vi "TLB Native Dynamic Events ver 0.06b.vi"() -> ()   [LabVIEW 2018]
uses:
  Labview Training Phase 2/Enum Controls/States for Action Engine.ctl
  Type def/TLB event states.ctl
  Type def/TLB MHL States.ctl
  <vilib>/Studica/Studica Toolkit/Background/I2C Channel.ctl
  <vilib>/Studica/Studica Toolkit/NavX/NavX.lvlib
  <vilib>/myRIO/Common/Instrument Driver Framework/myRIO v1.0/AI/typedefs/AI Channels Enum.ctl
  <vilib>/myRIO/Common/Instrument Driver Framework/myRIO v1.0/AI/typedefs/AI Channels List.ctl
  Type def/Type def.ctl
  Type def/Motor Control Cluster.ctl
  <vilib>/Studica/Studica Blackhawk/Blackhawk.lvlib
  <vilib>/vision/driver/NI_Vision_Acquisition_Software.lvlib
  <vilib>/userdefined/High Color/IMAQdx.ctl
  <vilib>/vision/driver/IMAQdx.llb/IMAQdx Buffer Number Mode.ctl
  <vilib>/vision/driver/IMAQdx.llb/IMAQdx Acquisition Mode.ctl
  Underlying VI's/Webcam FGV Low level ver/State control.ctl
  <vilib>/Studica/Studica Toolkit/Background/Mxp Selection.ctl
  <vilib>/ptbypt/NI_PtbyPt.lvlib
panel:
  out "Speed and distance cluster":T1
  out "error out":errorcluster
  out "Blackhawk loop":i32
  out "NavX Loop":i32
  out "Sensor Loop":i32
  out "User event loop":i32
  out "Event handling loop":i32
  out "Main Loop":i32
  out "Status loop":i32
  out "L/R average":fxp<+,64,64>
  out "Right Ultrasonic":fxp<+,64,16>
  out "Left Ultrasonic":fxp<+,64,16>
  out "Object detection count":T2
  out "Camera error":errorcluster
  out "Right IR Sensor":dbl
  out "Left IR Sensor":dbl
  in  "Servo Angle":u8(slide) scale=0.0..180.0
  in  "On/Off":bool
  out "Blackhawk error":errorcluster
  out "Value Read":bool
  out "Image Out":T3(plugin-control)
  out "element":T4
  out "Action Queue Items":i32
  out "State Logic Queue Items":i32
  out "Action Queues items":string[](array[string])=["Hardware reset", "Software reset", ""]
  out "State logic":T5=enum."Task 2"
  out "Action State":string
  in  "Tasks Selector":string(combo)="Default"
  out "Yaw":dbl
  out "NavX Info Out":T7
  out "LinearAcceleration":T8
  out "Displacement":T9
  out "YRPHfH":T10
  out "Object detected":bool
  in  "NavX Zero Yaw":bool
  in  "Return to IDLE":bool
  in  "Stop Queue":bool
  in  "Start Task":bool
  # "Camera Status Loop"
  # "TLB FRAMEWORK STATUS"
  # "Test Programme written by Calvin Loke    Dated: 28 Aug 2019\nTest Programme revised by Dr Alex See   Dated 30 Aug 2019\n\nProgramme version:   TLB Native Dynamic Events ver 0.04b.vi"
  # "Sequence of Actions"
  # "Continuous (Repeated)"
  # "Motor Control Loop"
  # "Sensor data"
  # "Blackhawk status"
  # "System Health Status Update"
  # "NAVX Control Loop"
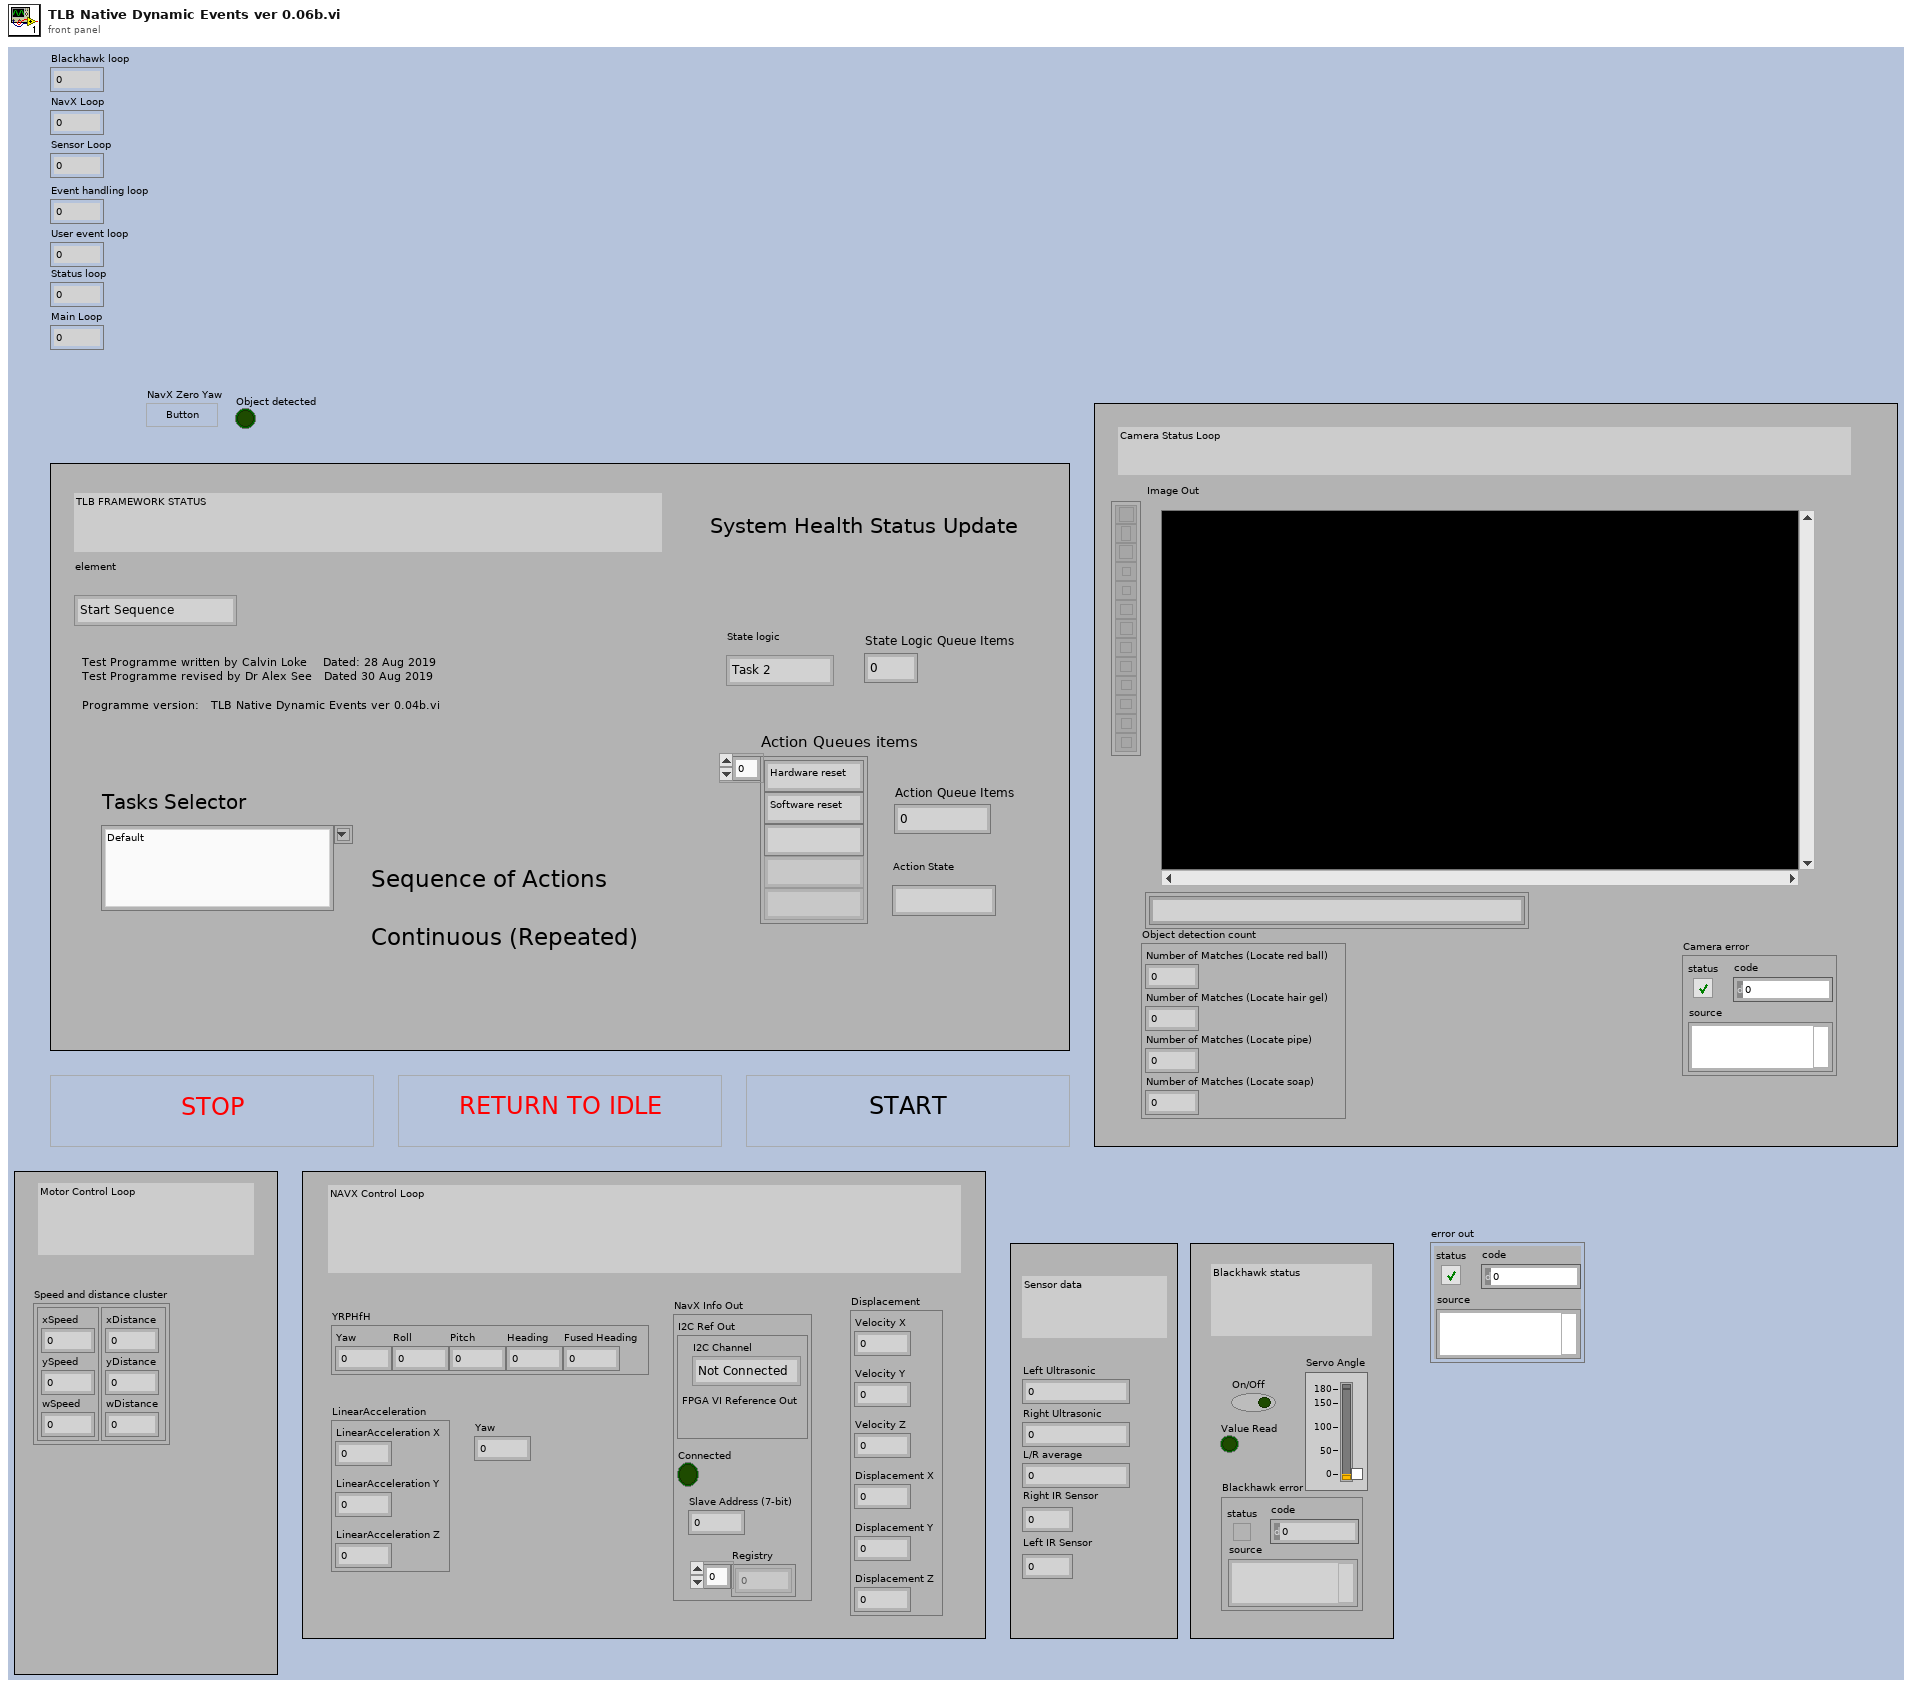
[diagram p1: front panel]
types:
  T1 = cluster{cluster{"xSpeed":dbl, "ySpeed":dbl, "wSpeed":dbl}, cluster{"xDistance":dbl, "yDistance":dbl, "wDistance":dbl}}
  T2 = cluster{"Number of Matches (Locate red ball)":i32, "Number of Matches (Locate hair gel)":i32, "Number of Matches (Locate pipe)":i32, "Number of Matches (Locate soap)":i32}
  T3 = typedef "IMAQ Image.ctl" = refnum<image>
  T4 = typedef "TLB event states.ctl" = enum16{"Start Sequence", "Exit", "Start Task 1", "Start Task 2", "Start Task 3", "Start Task 4", "Camera vision", "Wall follow mode", "Idle", "Start Drive Straight"}
  T5 = typedef "TLB MHL States.ctl" = enum16{"None", "Startup", "Idle", "Processing", "Shutdown", "Reset", "Task 1", "Task 2", "Task 3", "Task 4", "Task 4a", "Task 4b", "Task 4c", "Task 4d", "Task 4e", "Task 4f", "Task 4g", "Task 4h", "Acquire image", "Wall follow mode", "Autodrive", "Autodrive a"}
  T6 = typedef "I2C Channel.ctl" = enum16{"Not Connected", "A", "B"}
  T7 = cluster{"I2C Ref Out":cluster{"I2C Channel":T6, "FPGA VI Reference Out":refnum<k20>}, "Connected":bool, "Slave Address (7-bit)":u8, "Registry":u8[]}
  T8 = cluster{"LinearAcceleration X":dbl, "LinearAcceleration Y":dbl, "LinearAcceleration Z":dbl}
  T9 = cluster{"Velocity X":dbl, "Velocity Y":dbl, "Velocity Z":dbl, "Displacement X":dbl, "Displacement Y":dbl, "Displacement Z":dbl}
  T10 = cluster{"Yaw":dbl, "Roll":dbl, "Pitch":dbl, "Heading":dbl, "Fused Heading":dbl}
  T11 = typedef "States for Action Engine.ctl" = enum16{"Initialize", "Write", "Read"}
  T12 = typedef "Motor Control Cluster.ctl" = cluster{"Vx":dbl, "Vy":dbl, "Vw":dbl}
  T13 = typedef "Type def.ctl" = cluster{"Front Ultrasonic Obstruct":bool, "Left Ultrasonic Obstruct":bool, "Right Ultrasonic Obstruct ":bool}
  T14 = typedef "NI_Vision_Acquisition_Software.lvlib/IMAQdx Acquisition Mode.ctl" = enum32{"One Shot", "Continuous"}
  T15 = typedef "IMAQdx.ctl" = refnum<k21>
  T16 = typedef "NI_Vision_Acquisition_Software.lvlib/IMAQdx Buffer Number Mode.ctl" = enum32{"Next", "Last", "Buffer Number", "Every", "Last New"}
  T17 = typedef "Mxp Selection.ctl" = enum16{"MXP A", "MXP B"}
  T18 = cluster{"xTargetSpeed":dbl, "yTargetSpeed":dbl, "wTargetSpeed":dbl}
  T19 = typedef "State control.ctl" = enum16{"Initialise", "Start camera", "Continuous Acquisition ", "Stop camera", "Dispose all"}
  T20 = cluster{"xDistance":dbl, "yDistance":dbl, "wDistance":dbl}
  T21 = typedef "AI Channels List.ctl" = T22[]
  T22 = typedef "AI Channels Enum.ctl" = enum16{"Not Connected", "AudioIn/Left", "AudioIn/Right", "C/AI0", "C/AI1", "A/AI0", "A/AI1", "A/AI2", "A/AI3", "A/AI4", "A/AI5", "A/AI6", "A/AI7", "B/AI0", "B/AI1", "B/AI2", "B/AI3", "B/AI4", "B/AI5", "B/AI6", "B/AI7", "AI/AI0", "AI/AI1", "AI/AI2", "AI/AI3", "A/AI0 (DIFF)", "A/AI1 (DIFF)", "A/AI2 (DIFF)", "A/AI3 (DIFF)", "B/AI0 (DIFF)", "B/AI1 (DIFF)", "B/AI2 (DIFF)", "B/AI3 (DIFF)"}
  T23 = cluster{"I2C Channel":T6, "FPGA VI Reference Out":refnum<k20>}
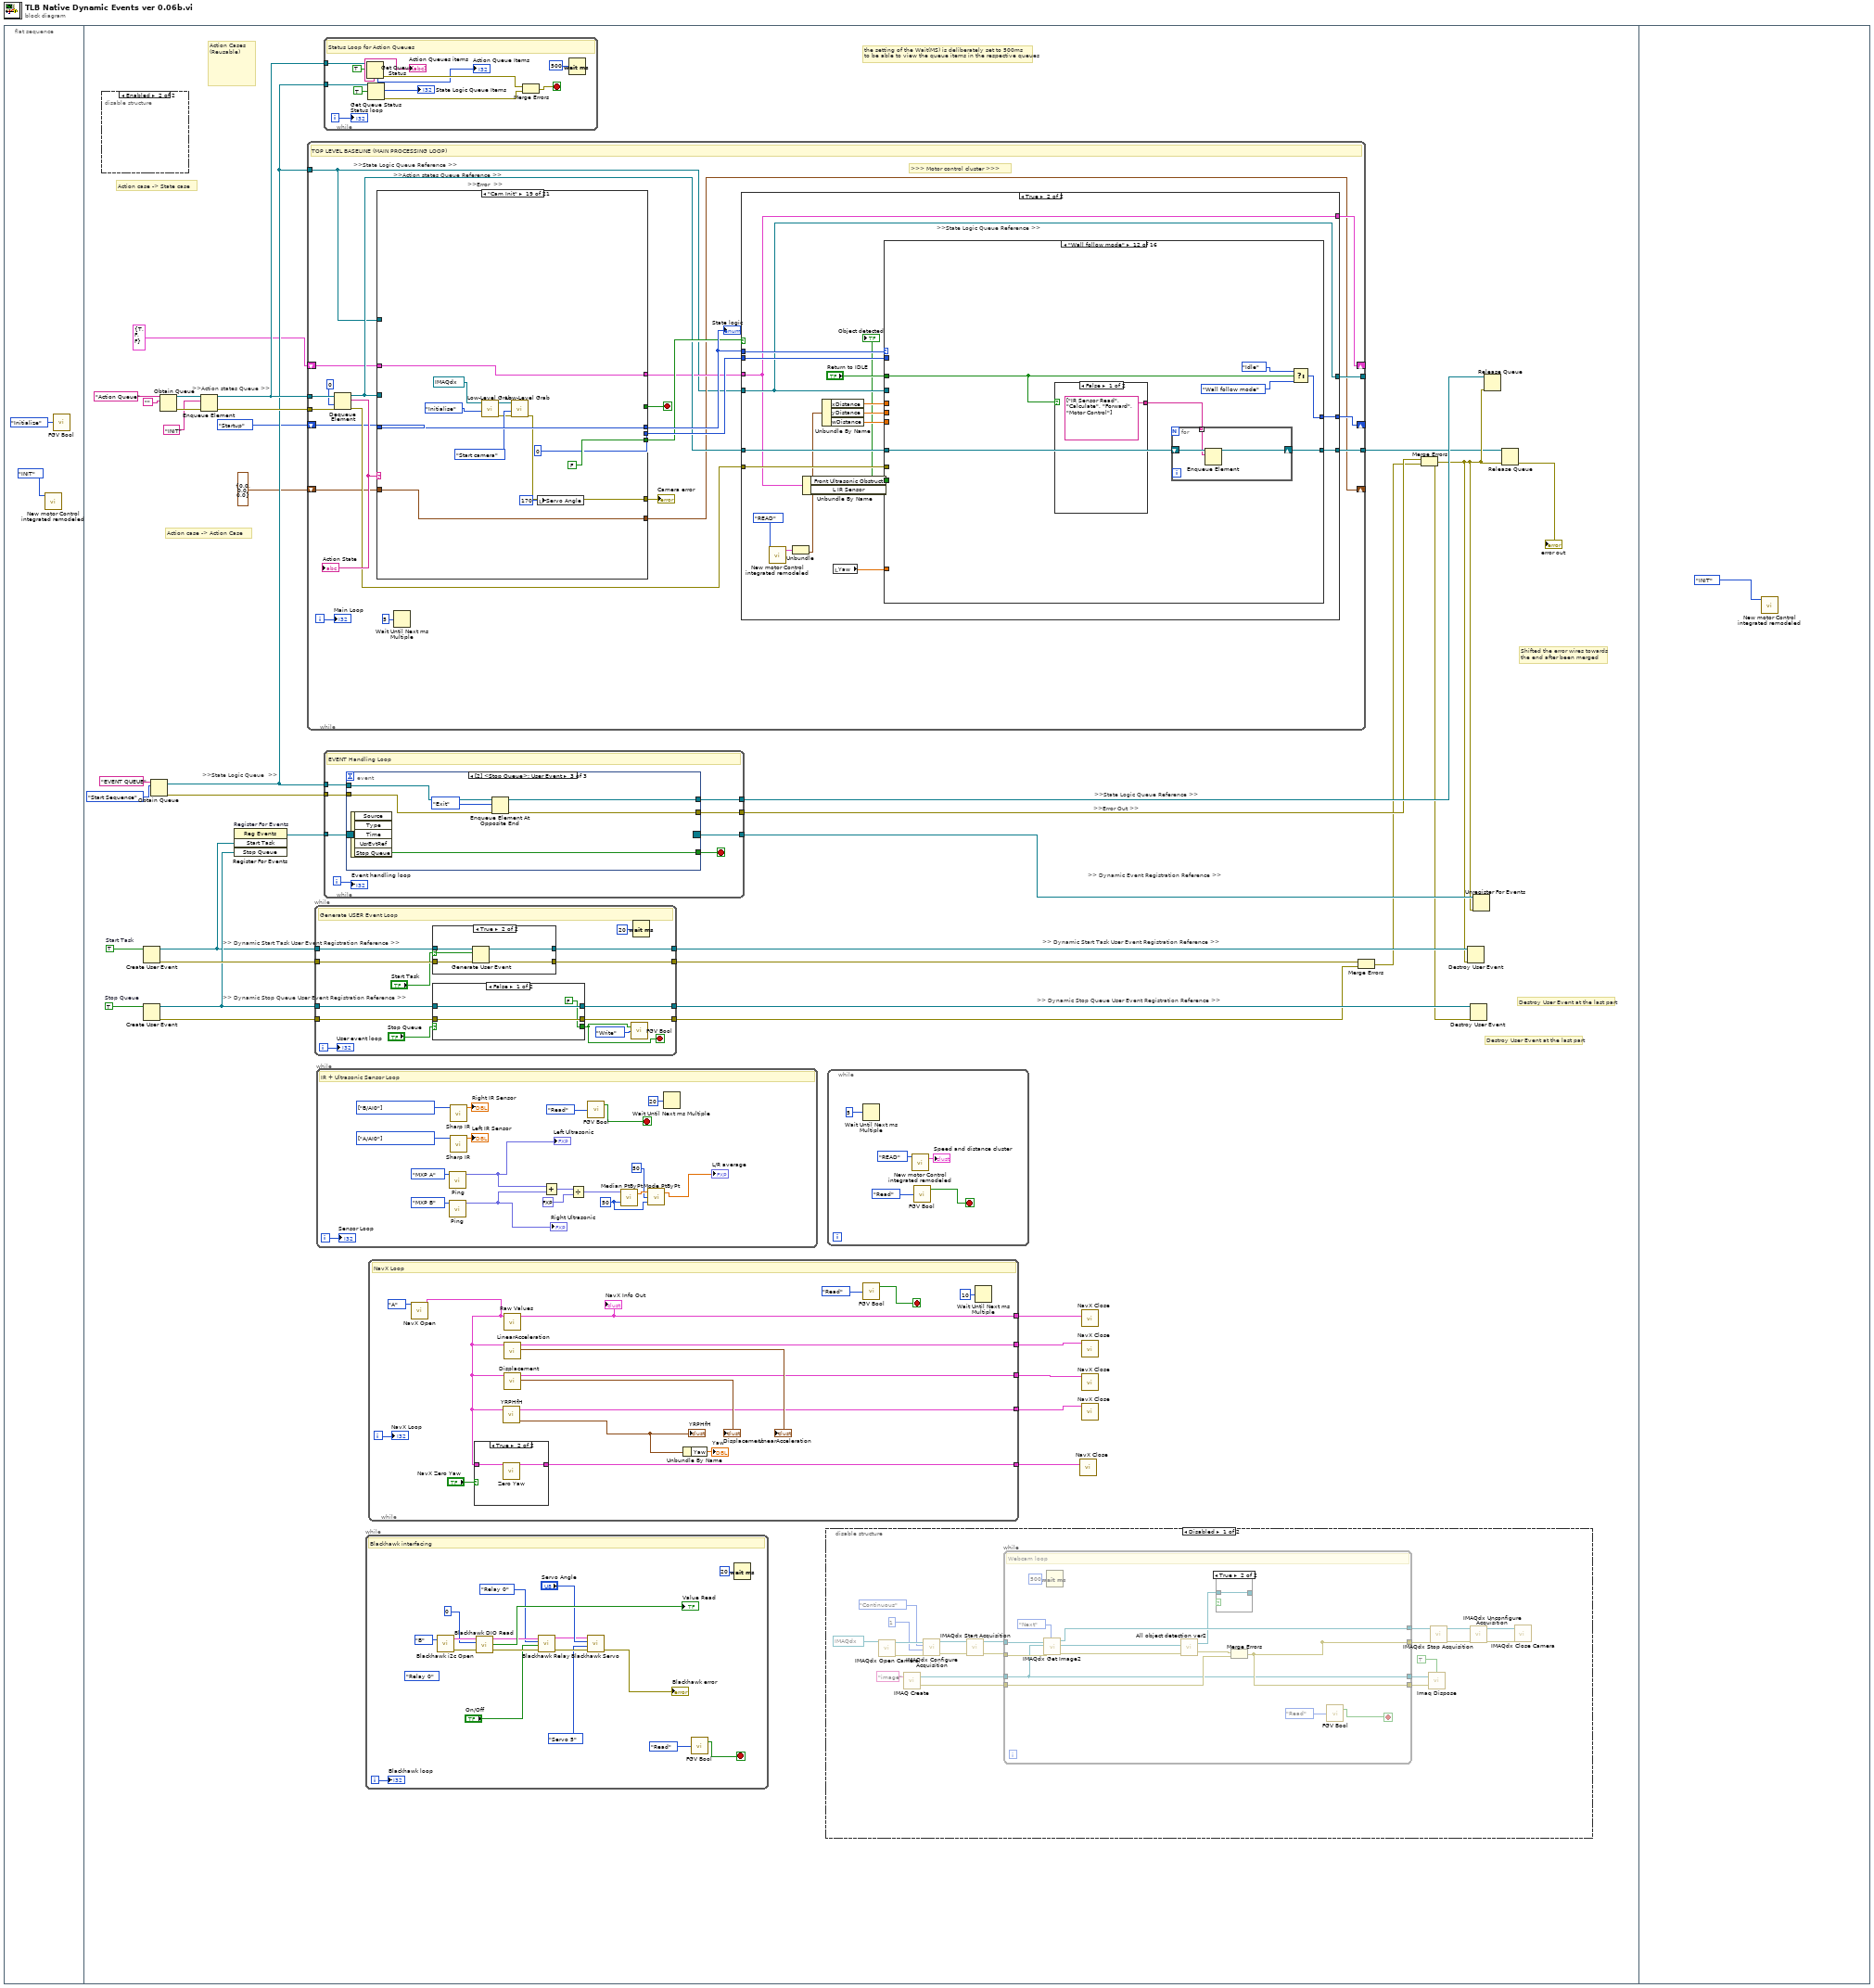
[diagram p0: block diagram]
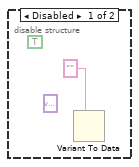
[diagram p5: hidden frame]
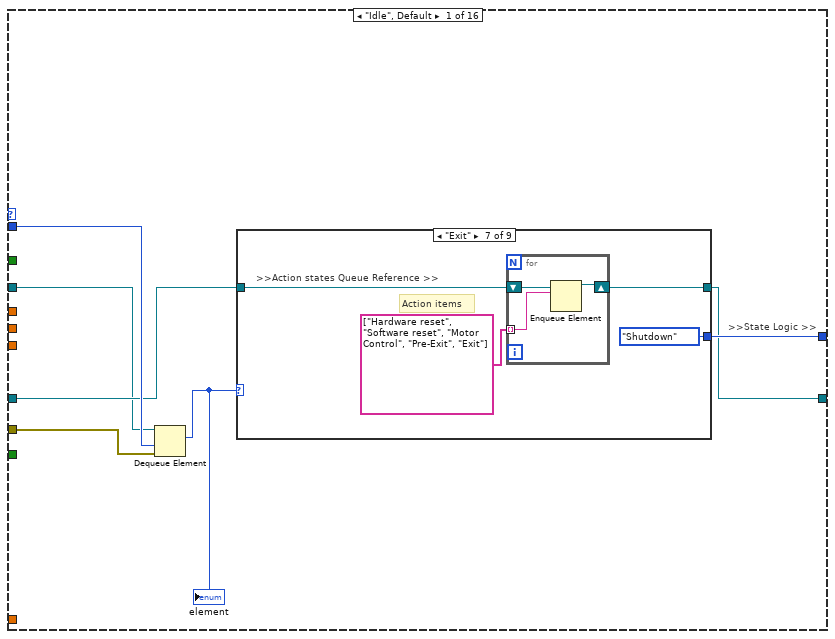
[diagram p7: hidden frame]
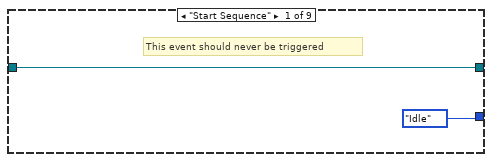
[diagram p8: hidden frame]
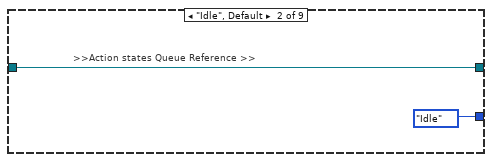
[diagram p9: hidden frame]
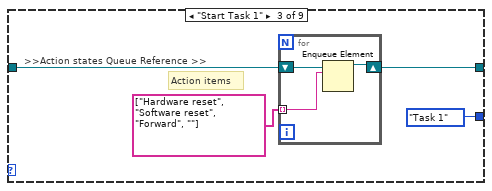
[diagram p10: hidden frame]
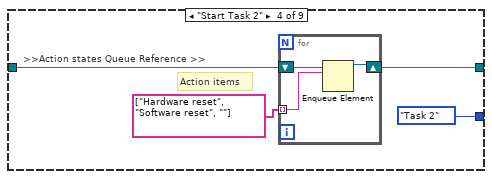
[diagram p11: hidden frame]
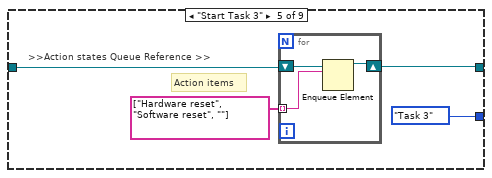
[diagram p12: hidden frame]
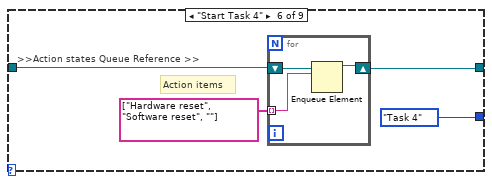
[diagram p13: hidden frame]
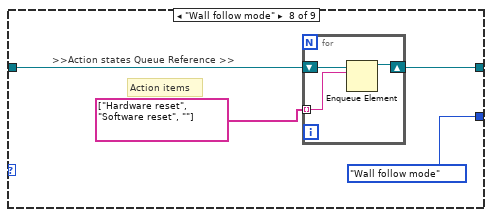
[diagram p14: hidden frame]
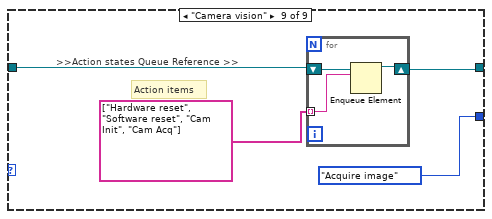
[diagram p15: hidden frame]
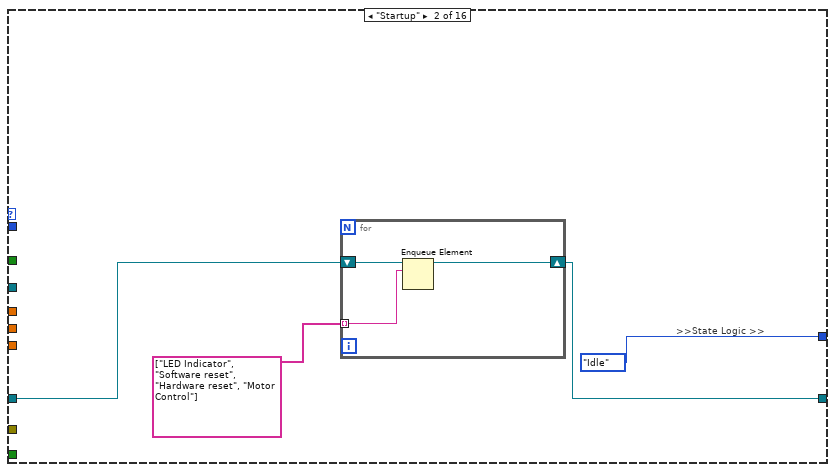
[diagram p16: hidden frame]
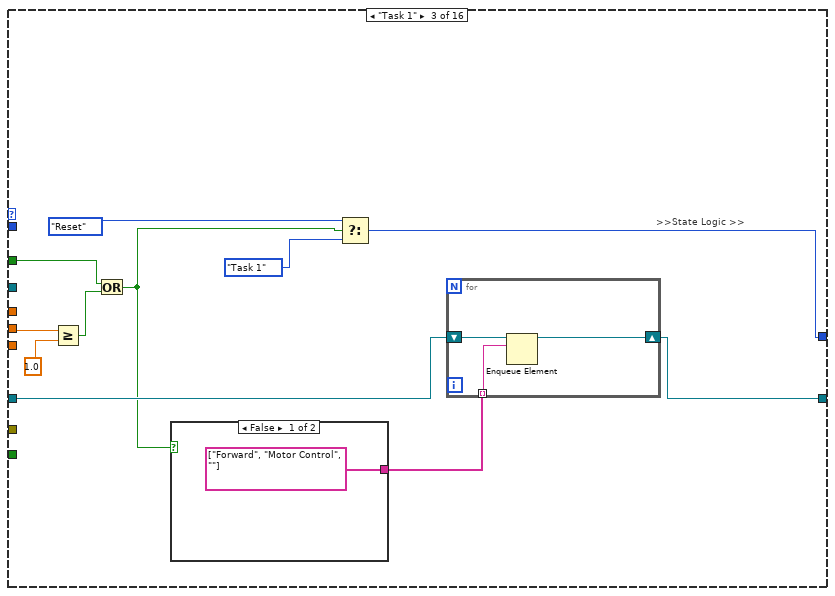
[diagram p17: hidden frame]
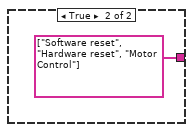
[diagram p18: hidden frame]
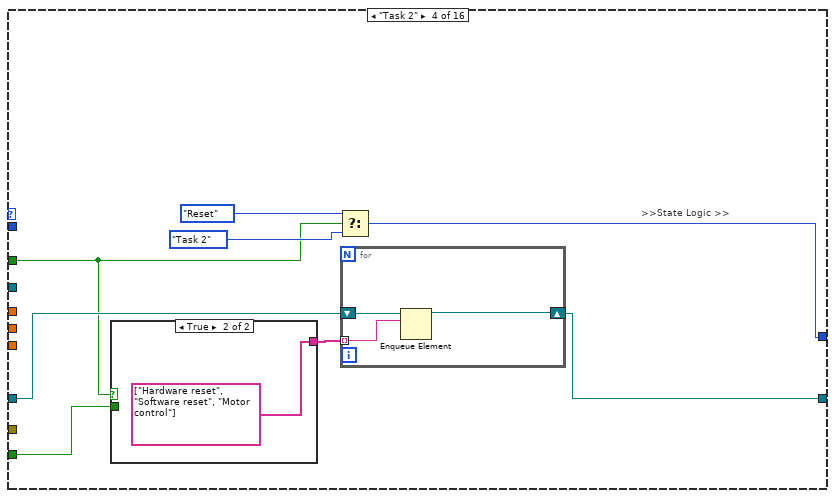
[diagram p19: hidden frame]
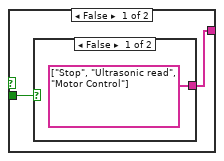
[diagram p20: hidden frame]
diagram:
  n1 = flat-sequence {
    frame #0 {
      n2 = call "New motor Control integrated remodeled.vi"("States"=enum16{"RESET ENCODER", "WRITE", "READ", "INIT"}."INIT") -> ()  [unwired: 4 in, 2 out]
      n3 = call "FGV Bool.vi"("Init/Read/Write State"=States_for_Action_Engine."Initialize") -> ()  [unwired: 2 in, 2 out]
    }
    frame #1 {
      w38 = TRUE  # Stop Queue
      w37 = TRUE  # Start Task
      # "Action case -> Action Case"
      # "Action case -> State case"
      # "the setting of the Wait(MS) is deliberately set to 500ms\nto be able to view the queue items in the respective queues"
      # "Action Cases\n(Reusable)"
      # ">>Error Out >>"
      # ">> Dynamic Stop Queue User Event Registration Reference >>"
      # ">> Dynamic Start Task User Event Registration Reference >>"
      # ">> Dynamic Stop Queue User Event Registration Reference >>"
      # ">> Dynamic Start Task User Event Registration Reference >>"
      # ">> Dynamic Event Registration Reference >>"
      # ">>Action states Queue >>"
      # ">>State Logic Queue  >>"
      # ">>State Logic Queue Reference >>"
      # "Destroy User Event at the last part"
      # "Destroy User Event at the last part"
      # "Shifted the error wires towards\nthe end after been merged"
      n4 = disable-structure shown="Enabled" {
        frame Disabled {
          (unwired) variant
          (unwired) TRUE
          n5 = Variant To Data(type="") -> ()  [unwired: 2 in, 2 out]
        }
        frame Enabled {
        }
      }
      n6 = Create User Event(user event datatype=w37) -> (user event=w29:refnum<user-event>, error out=w34:errorcluster)  [unwired: 1 in]
      n7 = Create User Event(user event datatype=w38) -> (user event=w30:refnum<user-event>, error out=w33:errorcluster)  [unwired: 1 in]
      n8 = Obtain Queue(name (unnamed)="EVENT QUEUE", element data type=TLB_event_states."Start Sequence" ("Enum")) -> (queue out=w14:refnum<queue>, error out=w20:errorcluster)  [unwired: 3 in, 1 out]
      n9 = Obtain Queue(name (unnamed)="Action Queue", element data type="") -> (queue out=w23:refnum<queue>, error out=w19:errorcluster)  [unwired: 3 in, 1 out]
      n10 = Enqueue Element(queue=w23, element="INIT", error in (no error)=w19) -> (queue out=w15:refnum<queue>, error out=w18:errorcluster)  [unwired: 1 in, 1 out]
      n11 = register-events "Register For Events"(w29, w30) -> (reference out=w28:refnum<event-registration>)  [unwired: 2 in, 1 out]
      n12 = while {
        tunnel: w14 -> [w151]
        shift-right: [w166] -> _
        shift-left: TLB_MHL_States."Startup" ("Enum") -> [w159]
        tunnel: w15 -> [w171]
        tunnel: w18 -> [w169]
        tunnel: [w168] -> _
        tunnel: [w167] -> w12
        shift-right: [w156] -> _
        shift-left: T13 {"Front Ultrasonic Obstruct"=TRUE, "Left Ultrasonic Obstruct"=FALSE, "Right Ultrasonic Obstruct "=FALSE} -> [w158]
        shift-right: [w154] -> _
        shift-left: T12 {"Vx"=0.0, "Vy"=0.0, "Vw"=0.0} -> [w155]
        i -> [w152]
        stop <- w164 stop-if-true
        # ">>> Motor control cluster >>>"
        # ">>Error  >>"
        # ">>Action states Queue Reference >>"
        # ">>State Logic Queue Reference >>"
        # "TOP LEVEL BASELINE (MAIN PROCESSING LOOP)"
        n13 = Dequeue Element(queue=w171, timeout in ms (-1)=0, error in (no error)=w169) -> (queue out=w160:refnum<queue>, element=w170:string, error out=w161:errorcluster)  [unwired: 1 out]
        "Action State" <- w170
        n14 = case shown="\"Cam Init\"" w170 {
          tunnel: [w419 w438 w443 w450 w458 w467 w475 w481 w491 w498 w504 w514 w524 TLB_MHL_States."Shutdown" ("Enum") w535 w545 w549 w563 w575 w584 w598] -> w172
          tunnel: [w426 0 0 0 0 0 0 0 0 0 0 0 0 0 0 0 0 0 0 0 0] -> w165
          tunnel: [_ _ _ _ _ _ _ _ _ _ _ _ _ TRUE _ _ _ _ _ _ _] -> w164
          tunnel: [TRUE FALSE FALSE FALSE FALSE FALSE FALSE FALSE FALSE FALSE FALSE FALSE FALSE FALSE FALSE FALSE FALSE FALSE FALSE FALSE FALSE] -> w163
          tunnel: w160 -> [w418 _ _ _ _ _ _ _ _ _ _ _ _ _ _ _ _ _ _ _ _]
          tunnel: w159 -> [w420 w438 w443 w450 w458 w467 w475 w481 w491 w498 w504 w514 w524 _ w535 w545 w549 w563 w575 w584 w598]
          tunnel: w158 -> [w424 w435 w440 w447 w455 w463 w471 w479 w487 w495 w505 w511 w520 w526 w536 w544 w552 w564 w576 w583 w594]
          tunnel: [w424 w435 w440 w447 w455 w463 w471 w479 w487 w495 w505 w510 w520 w526 w536 w541 w551 w564 w576 w583 w594] -> w157
          tunnel: w155 -> [w423 w434 w439 w445 w453 w461 w470 w477 w486 w493 w501 w508 w519 w525 w532 w538 w546 w555 w574 w587 w595]
          tunnel: [w423 w434 w439 w446 w454 w462 w469 w478 w485 w494 w501 w508 w517 w525 w532 w538 w546 w556 w574 w587 w595] -> w154
          tunnel: [_ _ _ _ _ _ _ _ _ _ _ _ _ _ _ _ _ _ w565 w579 w588] -> w153
          tunnel: w151 -> [w422 _ _ _ _ _ _ _ _ _ _ _ _ _ _ _ _ _ _ _ _]
          frame "No action", Default {
            n15 = Get Queue Status(queue=w422) -> (error out=w421:errorcluster)  [unwired: 2 in, 7 out]
            n16 = case shown="Error" w421 {
              tunnel: w420 -> [w427 _]
              tunnel: [w427 TLB_MHL_States."Shutdown" ("Enum")] -> w419
              tunnel: w418 -> [_ _]
              frame No Error {
              }
              frame Error {
                n17 = call "New motor Control integrated remodeled.vi"("States"=enum16{"RESET ENCODER", "WRITE", "READ", "INIT"}."WRITE", "Target Speed"=T18 {"xTargetSpeed"=0.0, "yTargetSpeed"=0.0, "wTargetSpeed"=0.0}) -> ()  [unwired: 3 in, 2 out]
              }
            }
            n18 = case shown="\"Startup\", Default" w420 {
              tunnel: [0 100] -> w426
              frame "Startup", Default {
              }
              frame "Idle" {
              }
            }
          }
          frame "Init" {
            # ">>State Logic  >>"
            n19 = local write "Servo Angle"(u8 90 ("Servo Angle")) -> ()
          }
          frame "LED Indicator" {
          }
          frame "Forward" {
            n20 = local write "NavX Zero Yaw"(FALSE ("NavX Zero Yaw")) -> ()
            n21 = Bundle By Name(cluster=w445, "Vy"=0.8) -> (w446:T12)
          }
          frame "Reverse" {
            n22 = local write "NavX Zero Yaw"(FALSE ("NavX Zero Yaw")) -> ()
            n23 = Bundle By Name(cluster=w453, "Vy"=-0.6) -> (w454:T12)
          }
          frame "Right" {
            n24 = local write "NavX Zero Yaw"(FALSE ("NavX Zero Yaw")) -> ()
            n25 = Bundle By Name(cluster=w461, "Vx"=0.6) -> (w462:T12)
          }
          frame "Left" {
            n26 = Bundle By Name(cluster=w470, "Vx"=-0.6) -> (w469:T12)
            n27 = local write "NavX Zero Yaw"(FALSE ("NavX Zero Yaw")) -> ()
          }
          frame "Rotate CW" {
            n28 = local write "NavX Zero Yaw"(FALSE ("NavX Zero Yaw")) -> ()
            n29 = Bundle By Name(cluster=w477, "Vw"=-0.3) -> (w478:T12)
          }
          frame "Rotate ACW" {
            n30 = local write "NavX Zero Yaw"(FALSE ("NavX Zero Yaw")) -> ()
            n31 = Bundle By Name(cluster=w486, "Vw"=0.15) -> (w485:T12)
          }
          frame "Stop" {
            w492 = 0.0
            n32 = local write "NavX Zero Yaw"(FALSE ("NavX Zero Yaw")) -> ()
            n33 = Bundle By Name(cluster=w493, "Vx"=w492, "Vy"=w492, "Vw"=w492) -> (w494:T12)
          }
          frame "Motor control" {
            # "Replace with FGV"
            n34 = call "New motor Control integrated remodeled.vi"("States"=enum16{"RESET ENCODER", "WRITE", "READ", "INIT"}."WRITE", "Target Speed"=w501) -> ()  [unwired: 3 in, 2 out]
          }
          frame "Software reset" {
            w509 = FALSE ("NavX Zero Yaw")
            n35 = Wait (ms)(milliseconds to wait=u32 20) -> ()  [unwired: 1 out]
            n36 = local write "NavX Zero Yaw"(w509) -> ()
            n37 = Bundle By Name(cluster=w511, "Front Ultrasonic Obstruct"=w509, "L IR Sensor"=0.0) -> (w510:T13)
          }
          frame "Hardware reset" {
            w518 = 0.0
            n38 = Wait (ms)(milliseconds to wait=u32 20) -> ()  [unwired: 1 out]
            n39 = local write "NavX Zero Yaw"(TRUE ("NavX Zero Yaw")) -> ()
            n40 = call "New motor Control integrated remodeled.vi"("States"=enum16{"RESET ENCODER", "WRITE", "READ", "INIT"}."RESET ENCODER") -> ()  [unwired: 4 in, 2 out]
            n41 = Bundle By Name(cluster=w519, "Vx"=w518, "Vy"=w518, "Vw"=w518) -> (w517:T12)
          }
          frame "Exit" {
          }
          frame "Pre-Exit" {
            n42 = call "New motor Control integrated remodeled.vi"("States"=enum16{"RESET ENCODER", "WRITE", "READ", "INIT"}."INIT") -> ()  [unwired: 4 in, 2 out]
          }
          frame "Ultrasonic read" {
            # "Object detection"
            n43 = local read "L/R average"() -> (w537:fxp<+,64,64>)
            n44 = Less Or Equal?(x=w537, y=35.0) -> (x <= y?=w539:bool)
            n45 = Bundle By Name(cluster=w544, "Front Ultrasonic Obstruct"=w539) -> (w541:T13)
          }
          frame "IR Sensor Read" {
            n46 = local read "Left IR Sensor"() -> (w550:dbl)
            n47 = Bundle By Name(cluster=w552, "L IR Sensor"=w550) -> (w551:T13)
          }
          frame "Calculate" {
            n48 = Unbundle By Name(w564) -> ("L IR Sensor"=w560:dbl)
            n49 = Subtract(x=w560, y=20.0) -> (x-y=w558:dbl)
            n50 = Multiply(x=w558, y=0.1) -> (x*y=w554:dbl)
            n51 = Bundle By Name(cluster=w555, "Vy"=0.2, "Vw"=w554) -> (w556:T12)
          }
          frame "Cam Init" {
            n52 = call "Low-Level Grab.vi"("States"=State_control."Initialise", "Session In"=T15 "cam1") -> ("error out"=w566:errorcluster, "Session Out"=w567:T15)  [unwired: 7 in, 1 out]
            n53 = call "Low-Level Grab.vi"("error in (no error)"=w566, "States"=State_control."Start camera", "Session In"=w567) -> ("error out"=w565:errorcluster)  [unwired: 6 in, 2 out]
            n54 = local write "Servo Angle"(u8 170 ("Servo Angle")) -> ()
          }
          frame "Cam Acq" {
            n55 = call "Low-Level Grab.vi"("States"=State_control."Continuous Acquisition ") -> ("error out"=w580:errorcluster, "Image Out"=w581:T3)  [unwired: 8 in, 1 out]
            n56 = call "All object detection ver2.vi"("Image In"=w581, "error in"=w580) -> ("Image Out"=→"Image Out":T3, "Object detection count"=→"Object detection count":T2, "error out"=w579:errorcluster)
          }
          frame "Cam Exit" {
            n57 = call "Low-Level Grab.vi"("States"=State_control."Stop camera") -> ("error out"=w589:errorcluster, "Session Out"=w591:T15)  [unwired: 8 in, 1 out]
            n58 = local write "Servo Angle"(u8 90 ("Servo Angle")) -> ()
            n59 = call "Low-Level Grab.vi"("error in (no error)"=w589, "States"=State_control."Dispose all", "Session In"=w591) -> ("error out"=w588:errorcluster)  [unwired: 6 in, 2 out]
          }
        }
        "State logic" <- w172
        "Camera error" <- w153
        n60 = Wait Until Next ms Multiple(millisecond multiple=u32 5) -> ()  [unwired: 1 out]
        n61 = case shown="True" w163 {
          tunnel: w172 -> [w175 w193]
          tunnel: w151 -> [w176 w187]
          tunnel: w160 -> [w174 w192]
          tunnel: [w176 w187] -> w168
          tunnel: [w174 w191] -> w167
          tunnel: [w175 w190] -> w166
          tunnel: w161 -> [_ w189]
          tunnel: w165 -> [_ w188]
          tunnel: w157 -> [w173 w180]
          tunnel: [w173 w180] -> w156
          frame False {
          }
          frame True {
            # ">>State Logic Queue Reference >>"
            n62 = call "New motor Control integrated remodeled.vi"("States"=enum16{"RESET ENCODER", "WRITE", "READ", "INIT"}."READ") -> ("Speed and distance cluster"=w179:T1)  [unwired: 4 in, 1 out]
            n63 = Unbundle(w179) -> (w178:T20)  [unwired: 1 out]
            n64 = Unbundle By Name(w180) -> ("Front Ultrasonic Obstruct"=w181:bool)  [unwired: 1 out]
            "Object detected" <- w181
            n65 = Unbundle By Name(w178) -> ("xDistance"=w183:dbl, "yDistance"=w185:dbl, "wDistance"=w184:dbl)
            n66 = local read "Yaw"() -> (w182:dbl)
            n67 = case shown="\"Wall follow mode\"" w193 {
              tunnel: w187 -> [w194 _ _ _ _ _ _ _ _ _ _ _ _ _ _ _]
              tunnel: w192 -> [w196 w255 w267 w280 w302 w311 w325 w340 w353 w366 w377 w385 w398 w407 w410 w416]
              tunnel: [w195 w254 w266 w281 w301 w312 w324 w339 w352 w365 w376 w386 w397 w407 w409 w416] -> w191
              tunnel: [w199 TLB_MHL_States."Idle" ("Enum") w269 w282 w298 w315 w327 w338 w354 w364 TLB_MHL_States."Idle" ("Enum") w388 w396 TLB_MHL_States."Reset" ("Enum") TLB_MHL_States."Shutdown" ("Enum") TLB_MHL_States."Reset" ("Enum")] -> w190
              tunnel: w189 -> [w197 _ _ _ _ _ _ _ _ _ _ _ _ _ _ _]
              tunnel: w188 -> [w198 _ _ _ _ _ _ _ _ _ _ _ _ _ _ _]
              tunnel: "Return to IDLE" -> [_ _ w264 w279 w296 _ _ _ _ _ _ w383 w395 _ _ _]
              tunnel: w185 -> [_ _ w261 _ _ _ _ w335 _ _ _ _ _ _ _ _]
              tunnel: w184 -> [_ _ _ _ w293 _ _ _ _ _ _ _ _ _ _ _]
              tunnel: w183 -> [_ _ _ _ _ _ w321 _ w349 _ _ _ _ _ _ _]
              tunnel: w182 -> [_ _ _ _ _ _ _ _ _ _ _ _ _ _ _ _]
              tunnel: w181 -> [_ _ _ w277 _ w309 _ _ _ w363 _ _ _ _ _ _]
              frame "Idle", Default {
                # ">>State Logic >>"
                n68 = Dequeue Element(queue=w194, timeout in ms (-1)=w198, error in (no error)=w197) -> (element=w200:T4)  [unwired: 3 out]
                "element" <- w200
                n69 = case shown="\"Exit\"" w200 {
                  tunnel: [TLB_MHL_States."Idle" ("Enum") TLB_MHL_States."Idle" ("Enum") TLB_MHL_States."Task 1" ("Enum") TLB_MHL_States."Task 2" ("Enum") TLB_MHL_States."Task 3" ("Enum") TLB_MHL_States."Task 4" ("Enum") TLB_MHL_States."Shutdown" ("Enum") TLB_MHL_States."Wall follow mode" ("Enum") TLB_MHL_States."Acquire image" ("Enum")] -> w199
                  tunnel: [w202 w203 w207 w212 w221 w227 w233 w240 w248] -> w195
                  tunnel: w196 -> [w202 w203 w205 w213 w222 w228 w234 w241 w249]
                  frame "Start Sequence" {
                    # "This event should never be triggered"
                  }
                  frame "Idle", Default {
                    # ">>Action states Queue Reference >>"
                  }
                  frame "Start Task 1" {
                    # ">>Action states Queue Reference >>"
                    # "Action items"
                    n70 = for {
                      shift-right: [w211] -> w207
                      shift-left: w205 -> [w210]
                      tunnel: string[] ["Hardware reset", "Software reset", "Forward", ""] -> [w209] mode=indexing
                      n71 = Enqueue Element(queue=w210, element=w209) -> (queue out=w211:refnum<queue>)  [unwired: 2 in, 2 out]
                    }
                  }
                  frame "Start Task 2" {
                    # ">>Action states Queue Reference >>"
                    # "Action items"
                    n72 = for {
                      shift-right: [w218] -> w212
                      shift-left: w213 -> [w217]
                      tunnel: string[] ["Hardware reset", "Software reset", ""] -> [w216] mode=indexing
                      n73 = Enqueue Element(queue=w217, element=w216) -> (queue out=w218:refnum<queue>)  [unwired: 2 in, 2 out]
                    }
                  }
                  frame "Start Task 3" {
                    # ">>Action states Queue Reference >>"
                    # "Action items"
                    n74 = for {
                      shift-right: [w225] -> w221
                      shift-left: w222 -> [w224]
                      tunnel: string[] ["Hardware reset", "Software reset", ""] -> [w223] mode=indexing
                      n75 = Enqueue Element(queue=w224, element=w223) -> (queue out=w225:refnum<queue>)  [unwired: 2 in, 2 out]
                    }
                  }
                  frame "Start Task 4" {
                    # ">>Action states Queue Reference >>"
                    # "Action items"
                    n76 = for {
                      shift-right: [w232] -> w227
                      shift-left: w228 -> [w231]
                      tunnel: string[] ["Hardware reset", "Software reset", ""] -> [w230] mode=indexing
                      n77 = Enqueue Element(queue=w231, element=w230) -> (queue out=w232:refnum<queue>)  [unwired: 2 in, 2 out]
                    }
                  }
                  frame "Exit" {
                    # ">>Action states Queue Reference >>"
                    # "Action items"
                    n78 = for {
                      shift-right: [w239] -> w233
                      shift-left: w234 -> [w238]
                      tunnel: string[] ["Hardware reset", "Software reset", "Motor Control", "Pre-Exit", "Exit"] -> [w237] mode=indexing
                      n79 = Enqueue Element(queue=w238, element=w237) -> (queue out=w239:refnum<queue>)  [unwired: 2 in, 2 out]
                    }
                  }
                  frame "Wall follow mode" {
                    # ">>Action states Queue Reference >>"
                    # "Action items"
                    n80 = for {
                      shift-right: [w246] -> w240
                      shift-left: w241 -> [w245]
                      tunnel: string[] ["Hardware reset", "Software reset", ""] -> [w244] mode=indexing
                      n81 = Enqueue Element(queue=w245, element=w244) -> (queue out=w246:refnum<queue>)  [unwired: 2 in, 2 out]
                    }
                  }
                  frame "Camera vision" {
                    # ">>Action states Queue Reference >>"
                    # "Action items"
                    n82 = for {
                      shift-right: [w253] -> w248
                      shift-left: w249 -> [w252]
                      tunnel: string[] ["Hardware reset", "Software reset", "Cam Init", "Cam Acq"] -> [w251] mode=indexing
                      n83 = Enqueue Element(queue=w252, element=w251) -> (queue out=w253:refnum<queue>)  [unwired: 2 in, 2 out]
                    }
                  }
                }
              }
              frame "Startup" {
                # ">>State Logic >>"
                n84 = for {
                  shift-right: [w259] -> w254
                  shift-left: w255 -> [w260]
                  tunnel: string[] ["LED Indicator", "Software reset", "Hardware reset", "Motor Control"] -> [w258] mode=indexing
                  n85 = Enqueue Element(queue=w260, element=w258) -> (queue out=w259:refnum<queue>)  [unwired: 2 in, 2 out]
                }
              }
              frame "Task 1" {
                # ">>State Logic >>"
                n86 = Greater Or Equal?(x=w261, y=1.0) -> (x >= y?=w262:bool)
                n87 = Or(x=w264, y=w262) -> (x .or. y?=w265:bool)
                n88 = case shown="False" w265 {
                  tunnel: [string[] ["Forward", "Motor Control", ""] string[] ["Software reset", "Hardware reset", "Motor Control"]] -> w268
                  frame False {
                  }
                  frame True {
                  }
                }
                n89 = Select(t=TLB_MHL_States."Reset" ("Enum"), s=w265, f=TLB_MHL_States."Task 1" ("Enum")) -> (s? t:f=w269:T5)
                n90 = for {
                  shift-right: [w275] -> w266
                  shift-left: w267 -> [w276]
                  tunnel: w268 -> [w274] mode=indexing
                  n91 = Enqueue Element(queue=w276, element=w274) -> (queue out=w275:refnum<queue>)  [unwired: 2 in, 2 out]
                }
              }
              frame "Task 2" {
                # ">>State Logic >>"
                n92 = case shown="True" w279 {
                  tunnel: [w286 string[] ["Hardware reset", "Software reset", "Motor control"]] -> w278
                  tunnel: w277 -> [w285 _]
                  frame False {
                    n93 = case shown="False" w285 {
                      tunnel: [string[] ["Stop", "Ultrasonic read", "Motor Control"] string[] ["Reverse", "Ultrasonic read", "Motor control"]] -> w286
                      frame False {
                      }
                      frame True {
                      }
                    }
                  }
                  frame True {
                  }
                }
                n94 = Select(t=TLB_MHL_States."Reset" ("Enum"), s=w279, f=TLB_MHL_States."Task 2" ("Enum")) -> (s? t:f=w282:T5)
                n95 = for {
                  shift-right: [w291] -> w281
                  shift-left: w280 -> [w292]
                  tunnel: w278 -> [w290] mode=indexing
                  n96 = Enqueue Element(queue=w292, element=w290) -> (queue out=w291:refnum<queue>)  [unwired: 2 in, 2 out]
                }
              }
              frame "Task 3" {
                n97 = Less Or Equal?(x=w293, y=-1.2) -> (x <= y?=w294:bool)
                n98 = Or(x=w294, y=w296) -> (x .or. y?=w297:bool)
                n99 = case shown="True" w297 {
                  tunnel: [string[] ["Rotate CW", "Motor Control"] string[] ["Software reset", "Hardware reset", "Motor Control"]] -> w303
                  frame False {
                  }
                  frame True {
                  }
                }
                n100 = for {
                  shift-right: [w305] -> w301
                  shift-left: w302 -> [w306]
                  tunnel: w303 -> [w304] mode=indexing
                  n101 = Enqueue Element(queue=w306, element=w304) -> (queue out=w305:refnum<queue>)  [unwired: 2 in, 2 out]
                }
                n102 = Select(t=TLB_MHL_States."Reset" ("Enum"), s=w297, f=TLB_MHL_States."Task 3" ("Enum")) -> (s? t:f=w298:T5)
              }
              frame "Task 4" {
                n103 = case shown="True" w309 {
                  tunnel: [string[] ["Forward", "Ultrasonic read", "Motor Control"] string[] ["Stop", "Hardware reset", "Software reset", "Motor Control"]] -> w310
                  frame False {
                  }
                  frame True {
                  }
                }
                n104 = for {
                  shift-right: [w319] -> w312
                  shift-left: w311 -> [w320]
                  tunnel: w310 -> [w318] mode=indexing
                  n105 = Enqueue Element(queue=w320, element=w318) -> (queue out=w319:refnum<queue>)  [unwired: 2 in, 2 out]
                }
                n106 = Select(t=TLB_MHL_States."Task 4a" ("Enum"), s=w309, f=TLB_MHL_States."Task 4" ("Enum")) -> (s? t:f=w315:T5)
              }
              frame "Task 4a" {
                n107 = Greater Or Equal?(x=w321, y=0.5) -> (x >= y?=w323:bool)
                n108 = case shown="True" w323 {
                  tunnel: [string[] ["Right", "Motor Control"] string[] ["Stop", "Hardware reset", "Software reset", "Motor Control"]] -> w326
                  frame False {
                  }
                  frame True {
                  }
                }
                n109 = for {
                  shift-right: [w333] -> w324
                  shift-left: w325 -> [w334]
                  tunnel: w326 -> [w332] mode=indexing
                  n110 = Enqueue Element(queue=w334, element=w332) -> (queue out=w333:refnum<queue>)  [unwired: 2 in, 2 out]
                }
                n111 = Select(t=TLB_MHL_States."Task 4b" ("Enum"), s=w323, f=TLB_MHL_States."Task 4a" ("Enum")) -> (s? t:f=w327:T5)
              }
              frame "Task 4b" {
                n112 = Greater Or Equal?(x=w335, y=0.75) -> (x >= y?=w336:bool)
                n113 = case shown="False" w336 {
                  tunnel: [string[] ["Forward", "Motor control"] string[] ["Stop", "Hardware reset", "Software reset"]] -> w341
                  frame False {
                  }
                  frame True {
                  }
                }
                n114 = for {
                  shift-right: [w347] -> w339
                  shift-left: w340 -> [w348]
                  tunnel: w341 -> [w346] mode=indexing
                  n115 = Enqueue Element(queue=w348, element=w346) -> (queue out=w347:refnum<queue>)  [unwired: 2 in, 2 out]
                }
                n116 = Select(t=TLB_MHL_States."Task 4c" ("Enum"), s=w336, f=TLB_MHL_States."Task 4b" ("Enum")) -> (s? t:f=w338:T5)
              }
              frame "Task 4c" {
                n117 = Less Or Equal?(x=w349, y=-0.65) -> (x <= y?=w350:bool)
                n118 = case shown="True" w350 {
                  tunnel: [string[] ["Left", "Motor Control"] string[] ["Stop", "Hardware reset", "Software reset", "Motor Control"]] -> w355
                  frame False {
                  }
                  frame True {
                  }
                }
                n119 = for {
                  shift-right: [w361] -> w352
                  shift-left: w353 -> [w362]
                  tunnel: w355 -> [w360] mode=indexing
                  n120 = Enqueue Element(queue=w362, element=w360) -> (queue out=w361:refnum<queue>)  [unwired: 2 in, 2 out]
                }
                n121 = Select(t=TLB_MHL_States."Task 4d" ("Enum"), s=w350, f=TLB_MHL_States."Task 4c" ("Enum")) -> (s? t:f=w354:T5)
              }
              frame "Task 4d" {
                n122 = case shown="True" w363 {
                  tunnel: [string[] ["Forward", "Ultrasonic Read", "Motor Control"] string[] ["Stop", "Hardware reset", "Software reset", "Motor Control"]] -> w367
                  frame False {
                  }
                  frame True {
                  }
                }
                n123 = for {
                  shift-right: [w373] -> w365
                  shift-left: w366 -> [w374]
                  tunnel: w367 -> [w372] mode=indexing
                  n124 = Enqueue Element(queue=w374, element=w372) -> (queue out=w373:refnum<queue>)  [unwired: 2 in, 2 out]
                }
                n125 = Select(t=TLB_MHL_States."Task 4e" ("Enum"), s=w363, f=TLB_MHL_States."Task 4d" ("Enum")) -> (s? t:f=w364:T5)
              }
              frame "Reset" {
                n126 = for {
                  shift-right: [w381] -> w376
                  shift-left: w377 -> [w382]
                  tunnel: string[] ["Software reset", "Hardware reset", ""] -> [w380] mode=indexing
                  n127 = Enqueue Element(queue=w382, element=w380) -> (queue out=w381:refnum<queue>)  [unwired: 2 in, 2 out]
                }
                n128 = Wait (ms)(milliseconds to wait=u32 250) -> ()  [unwired: 1 out]
              }
              frame "Wall follow mode" {
                n129 = case shown="False" w383 {
                  tunnel: [string[] ["IR Sensor Read", "Calculate", "Forward", "Motor Control"] string[] ["Hardware reset", "Software reset", "Motor Control"]] -> w384
                  frame False {
                  }
                  frame True {
                  }
                }
                n130 = for {
                  shift-right: [w393] -> w386
                  shift-left: w385 -> [w394]
                  tunnel: w384 -> [w392] mode=indexing
                  n131 = Enqueue Element(queue=w394, element=w392) -> (queue out=w393:refnum<queue>)  [unwired: 2 in, 2 out]
                }
                n132 = Select(t=TLB_MHL_States."Idle" ("Enum"), s=w383, f=TLB_MHL_States."Wall follow mode" ("Enum")) -> (s? t:f=w388:T5)
              }
              frame "Acquire image" {
                n133 = case shown="True" w395 {
                  tunnel: [string[] ["Cam Acq"] string[] ["Hardware reset", "Software reset", "Cam Exit", ""]] -> w399
                  frame False {
                  }
                  frame True {
                  }
                }
                n134 = for {
                  shift-right: [w405] -> w397
                  shift-left: w398 -> [w406]
                  tunnel: w399 -> [w404] mode=indexing
                  n135 = Enqueue Element(queue=w406, element=w404) -> (queue out=w405:refnum<queue>)  [unwired: 2 in, 2 out]
                }
                n136 = Select(t=TLB_MHL_States."Idle" ("Enum"), s=w395, f=TLB_MHL_States."Acquire image" ("Enum")) -> (s? t:f=w396:T5)
              }
              frame "Processing" {
              }
              frame "Shutdown" {
                # ">>State Logic >>"
                n137 = for {
                  shift-right: [w414] -> w409
                  shift-left: w410 -> [w415]
                  tunnel: string[] ["Software reset", "Hardware reset", "Motor Control", "Cam Exit", "Pre-Exit", "Exit"] -> [w413] mode=indexing
                  n138 = Enqueue Element(queue=w415, element=w413) -> (queue out=w414:refnum<queue>)  [unwired: 2 in, 2 out]
                }
              }
              frame "None" {
              }
            }
          }
        }
        "Main Loop" <- w152
      }
      n139 = while {
        tunnel: w29 -> [w645]
        tunnel: w30 -> [w644]
        tunnel: [w643] -> w36
        tunnel: [w642] -> w35
        tunnel: w34 -> [w641]
        tunnel: [w640] -> w32
        tunnel: w33 -> [w639]
        tunnel: [w638] -> w31
        i -> [w633]
        stop <- w634 stop-if-true
        # "Generate USER Event Loop"
        n140 = case shown="True" "Start Task" {
          selector: "Start Task" -> [_ w657]
          tunnel: w645 -> [w656 w661]
          tunnel: [w656 w660] -> w642
          tunnel: w641 -> [w655 w659]
          tunnel: [w655 w658] -> w640
          frame False {
          }
          frame True {
            n141 = Generate User Event(user event=w661, event data cluster=w657, error in=w659) -> (user event out=w660:refnum<user-event>, error out=w658:errorcluster)  [unwired: 1 in]
          }
        }
        n142 = case shown="False" "Stop Queue" {
          selector: "Stop Queue" -> [_ w650]
          tunnel: w644 -> [w649 w654]
          tunnel: [w649 w653] -> w643
          tunnel: w639 -> [w648 w652]
          tunnel: [w648 w651] -> w638
          tunnel: [FALSE w650] -> w634
          frame False {
          }
          frame True {
            n143 = Generate User Event(user event=w654, event data cluster=w650, error in=w652) -> (user event out=w653:refnum<user-event>, error out=w651:errorcluster)  [unwired: 1 in]
          }
        }
        n144 = call "FGV Bool.vi"("Init/Read/Write State"=States_for_Action_Engine."Write", "Input Node"=w634) -> ()  [unwired: 1 in, 2 out]
        n145 = Wait (ms)(milliseconds to wait=u32 20) -> ()  [unwired: 1 out]
        "User event loop" <- w633
      }
      n146 = while {
        i -> [w119]
        stop <- w131 stop-if-true
        w121 = 50 ("sample length")
        w136 = T21 [enum."A/AI0"] items=["Not Connected", "AudioIn/Left", "AudioIn/Right", "C/AI0", "C/AI1", "A/AI0", "A/AI1", "A/AI2", "A/AI3", "A/AI4", "A/AI5", "A/AI6", "A/AI7", "B/AI0", "B/AI1", "B/AI2", "B/AI3", "B/AI4", "B/AI5", "B/AI6", "B/AI7", "AI/AI0", "AI/AI1", "AI/AI2", "AI/AI3", "A/AI0 (DIFF)", "A/AI1 (DIFF)", "A/AI2 (DIFF)", "A/AI3 (DIFF)", "B/AI0 (DIFF)", "B/AI1 (DIFF)", "B/AI2 (DIFF)", "B/AI3 (DIFF)"] ("AI Channel")
        w137 = T21 [enum."B/AI0"] items=["Not Connected", "AudioIn/Left", "AudioIn/Right", "C/AI0", "C/AI1", "A/AI0", "A/AI1", "A/AI2", "A/AI3", "A/AI4", "A/AI5", "A/AI6", "A/AI7", "B/AI0", "B/AI1", "B/AI2", "B/AI3", "B/AI4", "B/AI5", "B/AI6", "B/AI7", "AI/AI0", "AI/AI1", "AI/AI2", "AI/AI3", "A/AI0 (DIFF)", "A/AI1 (DIFF)", "A/AI2 (DIFF)", "A/AI3 (DIFF)", "B/AI0 (DIFF)", "B/AI1 (DIFF)", "B/AI2 (DIFF)", "B/AI3 (DIFF)"] ("AI Channel")
        # "IR + Ultrasonic Sensor Loop"
        n147 = call <vilib>:"Ping.vi"("Mxp Side"=Mxp_Selection."MXP B") -> ("CM"=w125:fxp<+,64,16>)  [unwired: 8 in, 2 out]
        "Right Ultrasonic" <- w125
        n148 = call <vilib>:"Ping.vi"("Mxp Side"=Mxp_Selection."MXP A") -> ("CM"=w126:fxp<+,64,16>)  [unwired: 8 in, 2 out]
        "Left Ultrasonic" <- w126
        n149 = call <vilib>:"Sharp IR.vi"("AI Channel"=w137) -> ("Sharp IR Distance"=→"Right IR Sensor":dbl)  [unwired: 8 in, 2 out]
        n150 = call <vilib>:"Sharp IR.vi"("AI Channel"=w136) -> ("Sharp IR Distance"=→"Left IR Sensor":dbl)  [unwired: 8 in, 2 out]
        n151 = Add(x=w126, y=w125) -> (x+y=w128:fxp<+,64,17>)
        n152 = Divide(x=w128, y=fxp<+,64,17> 2.0) -> (x/y=w124:fxp<+,64,64>)
        n153 = call "FGV Bool.vi"("Init/Read/Write State"=States_for_Action_Engine."Read") -> ("Output node"=w131:bool)  [unwired: 2 in, 1 out]
        n154 = call <vilib>:"Median PtByPt.vi"("sample length"=w121, "x"=w124) -> ("median"=w123:dbl)  [unwired: 2 in, 1 out]
        n155 = call <vilib>:"Mode PtByPt.vi"("sample length"=w121, "intervals"=50, "x"=w123) -> ("mode"=→"L/R average":dbl)  [unwired: 1 in, 1 out]
        n156 = Wait Until Next ms Multiple(millisecond multiple=u32 20) -> ()  [unwired: 1 out]
        "Sensor Loop" <- w119
      }
      n157 = while {
        tunnel: w15 -> [w147]
        tunnel: w14 -> [w144]
        i -> [w138]
        stop <- w141 stop-if-true
        # "Status Loop for Action Queues"
        n158 = Get Queue Status(queue=w147, return elements? (F)=TRUE) -> (error out=w143:errorcluster, # elements in queue=→"Action Queue Items":i32, elements=→"Action Queues items":string[])  [unwired: 1 in, 5 out]
        n159 = Get Queue Status(queue=w144, return elements? (F)=TRUE) -> (# pending remove=→"State Logic Queue Items":i32, error out=w142:errorcluster)  [unwired: 1 in, 6 out]
        n160 = Merge Errors(w143, w142) -> (w141:errorcluster)
        n161 = Wait (ms)(milliseconds to wait=u32 500) -> ()  [unwired: 1 out]
        "Status loop" <- w138
      }
      n162 = while {
        tunnel: w28 -> [w606]
        tunnel: [w605] -> w27
        tunnel: w14 -> [w603]
        tunnel: [w602] -> w26
        tunnel: w20 -> [w601]
        tunnel: [w600] -> w17
        i -> [w599]
        stop <- w604 stop-if-true
        # "EVENT Handling Loop"
        n163 = event shown="[2] <Stop Queue>: User Event" {
          selector: w606 -> [_ _ _]
          dyn-events: [_ _ _] -> w605
          timeout: _ -> [_ _ _]
          tunnel: [FALSE FALSE w632] -> w604
          tunnel: w603 -> [w611 w618 w630]
          tunnel: [w610 w617 w631] -> w602
          tunnel: w601 -> [w608 w614 w628]
          tunnel: [w607 w613 w627] -> w600
          event Timeout {
            n164 = event-data() -> ()  [unwired: 1 in, 3 out]
            n165 = Enqueue Element(queue=w611, element=TLB_event_states."Idle" ("Enum"), error in (no error)=w608) -> (queue out=w610:refnum<queue>, error out=w607:errorcluster)  [unwired: 1 in, 1 out]
          }
          event User Event {
            n166 = event-data() -> ()  [unwired: 1 in, 5 out]
            n167 = case shown="\"RT Camera tracking\"" "Tasks Selector" {
              tunnel: [TLB_event_states."Idle" ("Enum") TLB_event_states."Start Task 1" ("Enum") TLB_event_states."Start Task 2" ("Enum") TLB_event_states."Start Task 3" ("Enum") TLB_event_states."Start Task 4" ("Enum") TLB_event_states."Wall follow mode" ("Enum") TLB_event_states."Camera vision" ("Enum")] -> w615
              frame Default {
              }
              frame "Task 1" {
              }
              frame "Task 2" {
              }
              frame "Task 3" {
              }
              frame "Task 4" {
              }
              frame "Wall following" {
              }
              frame "RT Camera tracking" {
              }
            }
            n168 = Enqueue Element(queue=w618, element=w615, error in (no error)=w614) -> (queue out=w617:refnum<queue>, error out=w613:errorcluster)  [unwired: 1 in, 1 out]
          }
          event User Event {
            n169 = event-data() -> ("Stop Queue"=w632:bool)  [unwired: 1 in, 4 out]
            n170 = Enqueue Element At Opposite End(queue=w630, element=TLB_event_states."Exit" ("Enum"), error in (no error)=w628) -> (queue out=w631:refnum<queue>, error out=w627:errorcluster)  [unwired: 1 in, 1 out]
          }
        }
        "Event handling loop" <- w599
      }
      n171 = while {
        i -> [w81]
        stop <- w92 stop-if-true
        (unwired) enum8{"Relay 0", "Relay 1", "Relay 2"}."Relay 0" ("Relay")
        # "Blackhawk interfacing"
        n172 = call <vilib>:"Blackhawk i2c Open.vi"("I2C Channel"=I2C_Channel."B") -> ("I2C Ref Out"=w98:T23, "error out"=w97:errorcluster)  [unwired: 2 in]
        n173 = call <vilib>:"Blackhawk DIO Read.vi"("I2C Ref In"=w98, "PIN"=u8 0, "error in (no error)"=w97) -> ("I2C Ref Out"=w90:T23, "Value Read"=→"Value Read":bool, "error out"=w91:errorcluster)  [unwired: 3 in]
        n174 = call <vilib>:"Blackhawk Relay.vi"("error in (no error)"=w91, "On/Off"="On/Off", "Relay"=enum8{"Relay 0", "Relay 1", "Relay 2"}."Relay 0", "I2C Ref In"=w90) -> ("error out"=w87:errorcluster, "I2C Ref Out"=w83:T23)  [unwired: 6 in]
        n175 = call <vilib>:"Blackhawk Servo.vi"("error in (no error)"=w87, "Servo Select"=enum16{"Servo 5", "Servo 6"}."Servo 5", "Servo Angle"="Servo Angle", "I2C Ref In"=w83) -> ("error out"=→"Blackhawk error":errorcluster)  [unwired: 6 in, 1 out]
        n176 = call "FGV Bool.vi"("Init/Read/Write State"=States_for_Action_Engine."Read") -> ("Output node"=w92:bool)  [unwired: 2 in, 1 out]
        n177 = Wait (ms)(milliseconds to wait=u32 20) -> ()  [unwired: 1 out]
        "Blackhawk loop" <- w81
      }
      n178 = while {
        tunnel: [w111] -> w8
        tunnel: [w108] -> w7
        tunnel: [w107] -> w5
        tunnel: [w106] -> w6
        tunnel: [w105] -> w4
        i -> [w99]
        stop <- w113 stop-if-true
        # "NavX Loop"
        n179 = call <vilib>:"NavX Open.vi"("I2C Channel"=I2C_Channel."A") -> ("NavX Info"=w100:T7)  [unwired: 9 in, 1 out]
        n180 = case shown="True" "NavX Zero Yaw" {
          tunnel: w100 -> [w115 w117]
          tunnel: [w115 w116] -> w105
          frame False {
          }
          frame True {
            n181 = call <vilib>:"Zero Yaw.vi"("NavX Info In"=w117) -> ("NavX Info Out"=w116:T7)  [unwired: 10 in]
          }
        }
        n182 = call <vilib>:"YRPHfH.vi"("NavX Info In"=w100) -> ("YRPHfH"=w103:T10, "NavX Info Out"=w107:T7)  [unwired: 3 in]
        "YRPHfH" <- w103
        n183 = call <vilib>:"Raw Values.vi"("NavX Info In"=w100) -> ("NavX Info Out"=w111:T7)  [unwired: 8 in, 1 out]
        "NavX Info Out" <- w111
        n184 = call <vilib>:"LinearAcceleration.vi"("NavX Info In"=w100) -> ("LinearAcceleration"=→"LinearAcceleration":T8, "NavX Info Out"=w108:T7)  [unwired: 9 in]
        n185 = call <vilib>:"Displacement.vi"("NavX Info In"=w100) -> ("Displacement"=→"Displacement":T9, "NavX Info Out"=w106:T7)  [unwired: 9 in]
        n186 = Unbundle By Name(w103) -> ("Yaw"=→"Yaw":dbl)
        n187 = call "FGV Bool.vi"("Init/Read/Write State"=States_for_Action_Engine."Read") -> ("Output node"=w113:bool)  [unwired: 2 in, 1 out]
        n188 = Wait Until Next ms Multiple(millisecond multiple=u32 10) -> ()  [unwired: 1 out]
        "NavX Loop" <- w99
      }
      n189 = disable-structure shown="Disabled" {
        frame Disabled {
          n190 = call <vilib>:"IMAQdx Open Camera.vi"("Session In"=T15 "cam1") -> ("error out"=w48:errorcluster, "Session Out"=w50:T15)  [unwired: 9 in]
          n191 = call "IMAQ Create"("Image Name"="image") -> ("New Image"=w63:T3, "error out"=w62:errorcluster)  [unwired: 4 in]
          n192 = call <vilib>:"IMAQdx Configure Acquisition.vi"("error in"=w48, "Number of Buffers"=u32 1, "Continuous?"=IMAQdx_Acquisition_Mode."Continuous", "Session In"=w50) -> ("error out"=w47:errorcluster, "Session Out"=w49:T15)  [unwired: 6 in]
          n193 = call <vilib>:"IMAQdx Start Acquisition.vi"("error in"=w47, "Session In"=w49) -> ("error out"=w57:errorcluster, "Session Out"=w58:T15)  [unwired: 8 in]
          n194 = while {
            tunnel: w63 -> [w72]
            tunnel: w62 -> [w76]
            tunnel: [w72] -> w61
            tunnel: [w75] -> w60
            tunnel: [w75] -> w52
            tunnel: w58 -> [w74]
            tunnel: w57 -> [w73]
            tunnel: [w70] -> w51
            stop <- w78 stop-if-true
            # "Webcam loop"
            n195 = call <vilib>:"IMAQdx Get Image2.vi"("Buffer Number Mode (Next)"=IMAQdx_Buffer_Number_Mode."Next", "error in"=w73, "Image In"=w72, "Session In"=w74) -> ("error out"=w67:errorcluster, "Image Out"=w68:T3, "Session Out"=w70:T15)  [unwired: 4 in, 1 out]
            n196 = Wait (ms)(milliseconds to wait=u32 500) -> ()  [unwired: 1 out]
            n197 = call "All object detection ver2.vi"("error in"=w67, "Image In"=w68) -> ("error out"=w69:errorcluster, "Image Out"=w65:T3)
            n198 = case shown="True" w66 {
              tunnel: [_ w80] -> _
              tunnel: w65 -> [_ w80]
              frame False {
              }
              frame True {
              }
            }
            n199 = Merge Errors(w69, w76) -> (w75:errorcluster)
            n200 = call "FGV Bool.vi"("Init/Read/Write State"=States_for_Action_Engine."Read") -> ("Output node"=w78:bool)  [unwired: 2 in, 1 out]
          }
          n201 = call "Imaq Dispose"("All Images? (No)"=TRUE, "Image"=w61, "error in (no error)"=w60) -> ()  [unwired: 3 in, 1 out]
          n202 = call <vilib>:"IMAQdx Stop Acquisition.vi"("error in"=w52, "Session In"=w51) -> ("error out"=w55:errorcluster, "Session Out"=w56:T15)  [unwired: 8 in]
          n203 = call <vilib>:"IMAQdx Unconfigure Acquisition.vi"("error in"=w55, "Session In"=w56) -> ("error out"=w53:errorcluster, "Session Out"=w54:T15)  [unwired: 8 in]
          n204 = call <vilib>:"IMAQdx Close Camera.vi"("error in"=w53, "Session In"=w54) -> ()  [unwired: 9 in, 1 out]
        }
        frame Enabled {
        }
      }
      n205 = while {
        stop <- w41 stop-if-true
        n206 = Wait Until Next ms Multiple(millisecond multiple=u32 5) -> ()  [unwired: 1 out]
        n207 = call "New motor Control integrated remodeled.vi"("States"=enum16{"RESET ENCODER", "WRITE", "READ", "INIT"}."READ") -> ("Speed and distance cluster"=→"Speed and distance cluster":T1)  [unwired: 4 in, 1 out]
        n208 = call "FGV Bool.vi"("Init/Read/Write State"=States_for_Action_Engine."Read") -> ("Output node"=w41:bool)  [unwired: 2 in, 1 out]
      }
      n209 = call <vilib>:"NavX Close.vi"("NavX Info In"=w4) -> ()  [unwired: 10 in, 1 out]
      n210 = call <vilib>:"NavX Close.vi"("NavX Info In"=w8) -> ()  [unwired: 10 in, 1 out]
      n211 = call <vilib>:"NavX Close.vi"("NavX Info In"=w7) -> ()  [unwired: 10 in, 1 out]
      n212 = call <vilib>:"NavX Close.vi"("NavX Info In"=w6) -> ()  [unwired: 10 in, 1 out]
      n213 = call <vilib>:"NavX Close.vi"("NavX Info In"=w5) -> ()  [unwired: 10 in, 1 out]
      n214 = Merge Errors "Merge Errors"(w32, w31) -> (w11:errorcluster)
      n215 = Merge Errors(w17, w11) -> (w13:errorcluster)
      "error out" <- w13
      n216 = Destroy User Event(user event=w35, error in=w13) -> ()  [unwired: 1 out]
      n217 = Destroy User Event(user event=w36, error in=w13) -> ()  [unwired: 1 out]
      n218 = Unregister For Events(event registration refnum=w27, error in=w13) -> ()  [unwired: 1 out]
      n219 = Release Queue(queue=w26, error in (no error)=w13) -> ()  [unwired: 1 in, 3 out]
      n220 = Release Queue(queue=w12, error in (no error)=w13) -> ()  [unwired: 1 in, 3 out]
    }
    frame #2 {
      n221 = call "New motor Control integrated remodeled.vi"("States"=enum16{"RESET ENCODER", "WRITE", "READ", "INIT"}."INIT") -> ()  [unwired: 4 in, 2 out]
    }
  }
